vi "closeHookViReference.vi"(8 "error in (no error)":errorcluster, 11 "TestSuite in":refnum<class "TestSuite.lvclass">) -> (0 "error out":errorcluster, 3 "TestSuite out":refnum<class "TestSuite.lvclass">)   [LabVIEW 2013, in "TestSuite.lvclass"]
uses:
  TestSuite.lvclass
  TestSuite.lvclass/TestSuite.ctl
panel:
  # "JKI VI Tester for LabVIEW\nhttp://jkisoft.com/vi-tester\nCopyright (C) 2007-2009, JKI <info@jkisoft.com>\nALL RIGHTS RESERVED"
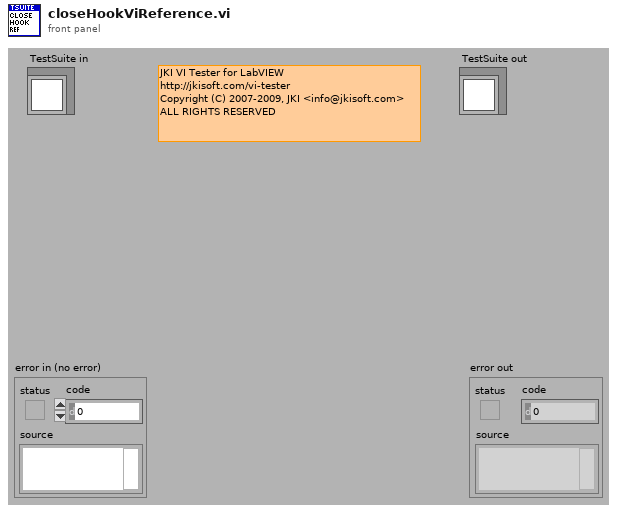
[diagram p1: front panel]
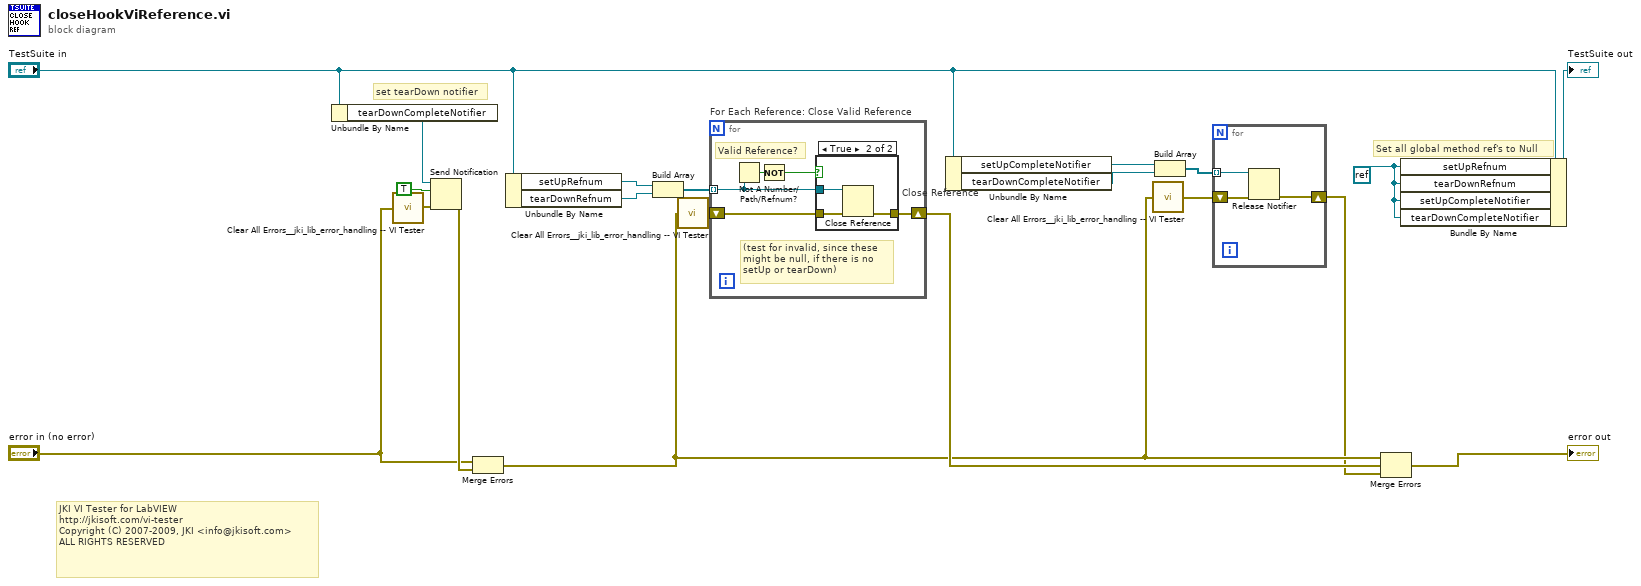
[diagram p0: block diagram]
diagram:
  w1 = refnum<k0> refnum
  # "JKI VI Tester for LabVIEW\nhttp://jkisoft.com/vi-tester\nCopyright (C) 2007-2009, JKI <info@jkisoft.com>\nALL RIGHTS RESERVED"
  # "set tearDown notifier"
  # "Set all global method ref's to Null"
  n1 = Unbundle By Name("TestSuite in") -> ("tearDownCompleteNotifier"=w5:refnum<notifier>)
  n2 = call "Clear All Errors__jki_lib_error_handling -- VI Tester.vi"("error in"="error in (no error)") -> ("no error out"=w3:errorcluster)  [unwired: 4 in]
  n3 = Send Notification(notification=TRUE, notifier=w5, error in (no error)=w3) -> (error out=w4:errorcluster)  [unwired: 1 out]
  n4 = Merge Errors("error in (no error)", w4) -> (w10:errorcluster)
  n5 = Unbundle By Name("TestSuite in") -> ("setUpRefnum"=w19:refnum<vi>, "tearDownRefnum"=w18:refnum<vi>)
  n6 = Build Array(w19, w18) -> (w16:refnum<vi>[])
  n7 = call "Clear All Errors__jki_lib_error_handling -- VI Tester.vi"("error in"=w10) -> ("no error out"=w17:errorcluster)  [unwired: 4 in]
  n8 = for "For Each Reference: Close Valid Reference" {
    shift-right: [w24] -> w15
    shift-left: w17 -> [w25]
    tunnel: w16 -> [w22] mode=indexing
    # "(test for invalid, since these might be null, if there is no setUp or tearDown)"
    # "Valid Reference?"
    n9 = Not A Number/Path/Refnum?(number/path/refnum=w22) -> (NaN/Path/Refnum?=w23:bool)
    n10 = Not(x=w23) -> (.not. x?=w21:bool)
    n11 = case "Close Reference" shown="True" w21 {
      tunnel: w25 -> [w26 w29]
      tunnel: w22 -> [_ w28]
      tunnel: [w26 w27] -> w24
      frame False {
      }
      frame True {
        n12 = Close Reference(reference=w28, error in (no error)=w29) -> (error out=w27:errorcluster)
      }
    }
  }
  n13 = Unbundle By Name("TestSuite in") -> ("setUpCompleteNotifier"=w13:refnum<notifier>, "tearDownCompleteNotifier"=w12:refnum<notifier>)
  n14 = call "Clear All Errors__jki_lib_error_handling -- VI Tester.vi"("error in"=w10) -> ("no error out"=w9:errorcluster)  [unwired: 4 in]
  n15 = Build Array(w13, w12) -> (w11:refnum<notifier>[])
  n16 = for {
    tunnel: w11 -> [w32] mode=indexing
    shift-right: [w31] -> w8
    shift-left: w9 -> [w30]
    n17 = Release Notifier(notifier=w32, error in (no error)=w30) -> (error out=w31:errorcluster)  [unwired: 1 in, 2 out]
  }
  n18 = Merge Errors(w10, w15, w8) -> (→"error out":errorcluster)
  n19 = Bundle By Name(cluster="TestSuite in", "setUpRefnum"=w1, "tearDownRefnum"=w1, "setUpCompleteNotifier"=w1, "tearDownCompleteNotifier"=w1) -> (→"TestSuite out":refnum<class "TestSuite.lvclass">)
